vi "Read Delimiters.vi"(8 "Error In":errorcluster, 11 "Node In":refnum<class "Abstract.lvclass">) -> (0 "Error Out":errorcluster, 2 "Delimiters":T1, 3 "Node Out":refnum<class "Abstract.lvclass">)   [LabVIEW 2018, in "Toolkit.lvlib" / "Nodes.lvlib" / "Abstract.lvclass"]
doc: "Gets the opening and closing components that surround, or delimit, a Mustache tag."
uses:
  Abstract.lvclass
  Type Definitions/Delimiters.ctl
  Abstract.lvclass/Abstract.ctl
  Toolkit.lvlib
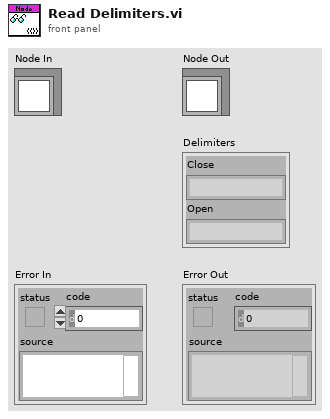
[diagram p1: front panel]
types:
  T1 = typedef "Toolkit.lvlib/Delimiters.ctl" = cluster{"Close":string, "Open":string}
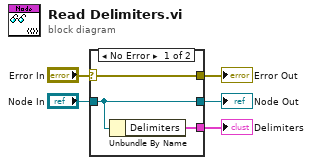
[diagram p0: block diagram]
diagram:
  n1 = case shown="No Error" "Error In" {
    selector: "Error In" -> [w8 w9]
    tunnel: [w8 w9] -> w4
    tunnel: [w7 w10] -> w2
    tunnel: "Node In" -> [w7 w10]
    tunnel: [w6 _] -> w1
    frame No Error {
      n2 = Unbundle By Name(w7) -> ("Delimiters"=w6:T1)
    }
    frame Error {
    }
  }
  "Error Out" <- w4
  "Node Out" <- w2
  "Delimiters" <- w1
